vi "Initialize Front Panel.vi"(8 "error in (no error)":errorcluster, 11 "Main ViewManager in":refnum<class "Splash Screen ViewManager.lvclass">) -> (0 "error out":errorcluster, 3 "Main ViewManager out":refnum<class "Splash Screen ViewManager.lvclass">)   [LabVIEW 2019, in "Splash Screen ViewManager.lvclass"]
doc: "<License>\nCopyright © 2017 Composed Systems, LLC | All rights reserved\nwww.composed.io\n\nAuthor: Ethan Stern <ethan.stern@composed.io>\n\nThis software is provided \"AS IS\" WITHOUT WARRANTIES, either express or implied, AND IS FOR EDUCATIONAL PURPOSES ONLY.\n</License>"
uses:
  <vilib>/gpm_packages/@cs/Car-wash/Source/Splash Screen ViewManager/Splash Screen ViewManager.lvclass
  <vilib>/gpm_packages/@cs/mva-viewable/Source/IViewManager/IViewManager/IViewManager.lvclass
  <vilib>/gpm_packages/@cs/mva-viewable/Source/IViewable/IViewable Messages/Insert Front Panel Msg/Insert Front Panel Msg.lvclass
  C:/Program Files/National Instruments/LabVIEW 2019/vi.lib/gpm_packages/@cs/mva-viewable/Source/IViewManager/IViewManager/IViewManager.lvclass
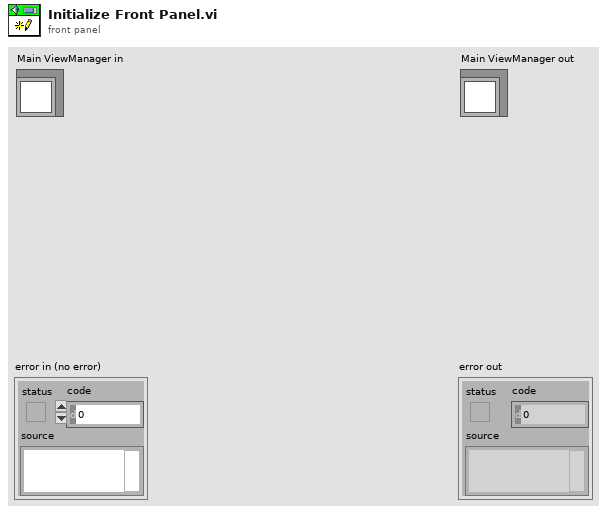
[diagram p1: front panel]
types:
  T1 = typedef "IViewable.lvlib/ProtectedSubpanel.lvclass/Protected Subpanel Reference.ctl" = refnum<data-value>
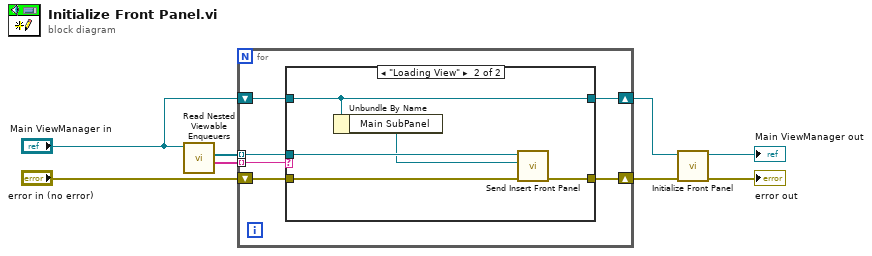
[diagram p0: block diagram]
diagram:
  n1 = call <vilib>:"Read Nested Viewable Enqueuers.vi"("IViewManager in"="Main ViewManager in") -> ("Viewable Names"=w7:string[], "Nested Viewable Enqueuers"=w8:refnum<class "Message Enqueuer.lvclass">[])  [unwired: 9 in]
  n2 = for {
    tunnel: w8 -> [w12] mode=indexing
    tunnel: w7 -> [w9] mode=indexing
    shift-right: [w10] -> w1
    shift-left: "Main ViewManager in" -> [w11]
    shift-right: [w13] -> w4
    shift-left: "error in (no error)" -> [w14]
    n3 = case shown="\"Loading View\"" w9 {
      tunnel: w14 -> [w15 w21]
      tunnel: [w15 w20] -> w13
      tunnel: w12 -> [_ w19]
      tunnel: [w16 w18] -> w10
      tunnel: w11 -> [w16 w18]
      frame Default {
      }
      frame "Loading View" {
        n4 = Unbundle By Name(w18) -> ("Main SubPanel"=w17:T1)
        n5 = call <vilib>:"Send Insert Front Panel.vi"("error in (no error)"=w21, "Protected Subpanel"=w17, "Message Enqueuer"=w19) -> ("error out"=w20:errorcluster)  [unwired: 7 in, 1 out]
      }
    }
  }
  n6 = call-parent "Initialize Front Panel.vi"("error in (no error)"=w4, "IViewable in"=w1) -> ("error out"=→"error out":errorcluster, "IViewable out"=→"Main ViewManager out":refnum<class "Splash Screen ViewManager.lvclass">)  [unwired: 8 in]
